vi "Decide Runtime Action.vi"(11 "Sequence Control":T1) -> (1 "Enum":T2)   [LabVIEW 2015, in "Sequencer Module runtime.lvclass"]
uses:
  Sequencer Module runtime.lvclass
  Sequencer Run Actions.ctl
  Sequencer Control.ctl
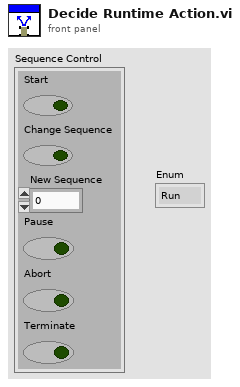
[diagram p1: front panel]
types:
  T1 = typedef "Sequencer Module runtime.lvclass/Sequencer Control.ctl" = cluster{"Start":bool, "Change Sequence":bool, "New Sequence":i32, "Pause":bool, "Abort":bool, "Terminate":bool}
  T2 = typedef "Sequencer Run Actions.ctl" = enum16{"Run", "Abort", "Pause", "Terminate"}
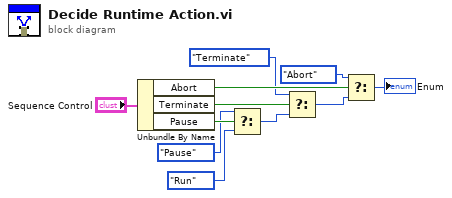
[diagram p0: block diagram]
diagram:
  n1 = Unbundle By Name("Sequence Control") -> ("Abort"=w5:bool, "Terminate"=w7:bool, "Pause"=w9:bool)
  n2 = Select(t=Sequencer_Run_Actions."Pause", s=w9, f=Sequencer_Run_Actions."Run") -> (s? t:f=w8:T2)
  n3 = Select(t=Sequencer_Run_Actions."Terminate", s=w7, f=w8) -> (s? t:f=w6:T2)
  n4 = Select(t=Sequencer_Run_Actions."Abort", s=w5, f=w6) -> (s? t:f=→"Enum":T2)
